vi "Build LV Spec.vi"() -> ()   [LabVIEW 2014]
doc: "This VI will execute a LabVIEW build spec.\n\nArguments:\nLabVIEW project file path\nLabVIEW build spec name\nBuild number"
uses:
  <userlib>/_OpenG.lib/file/file.llb/Convert File Extension (Path)__ogtk.vi
  <vilib>/AppBuilder/AB_API_Simple/Get Build Specification Version (path).vi
  <vilib>/AppBuilder/AB_API_Simple/Set Build Specification Version (path).vi
  <vilib>/AppBuilder/AB_API_Simple/Build (path).vi
  <vilib>/Wiresmith Technology/LabVIEW CLI/CLI Class/CLI.lvclass
  <vilib>/AppBuilder/AB_API_Simple/NI_App_Builder_API.lvlib
panel:
  out "error out":errorcluster
  out "Build Output":path[](array[path])
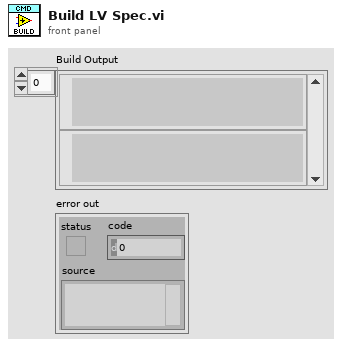
[diagram p1: front panel]
types:
  T1 = typedef "NI_App_Builder_API.lvlib/Build Specification Version.ctl" = cluster{"Major":u16, "Minor":u16, "Fix":u16, "Build":u16}
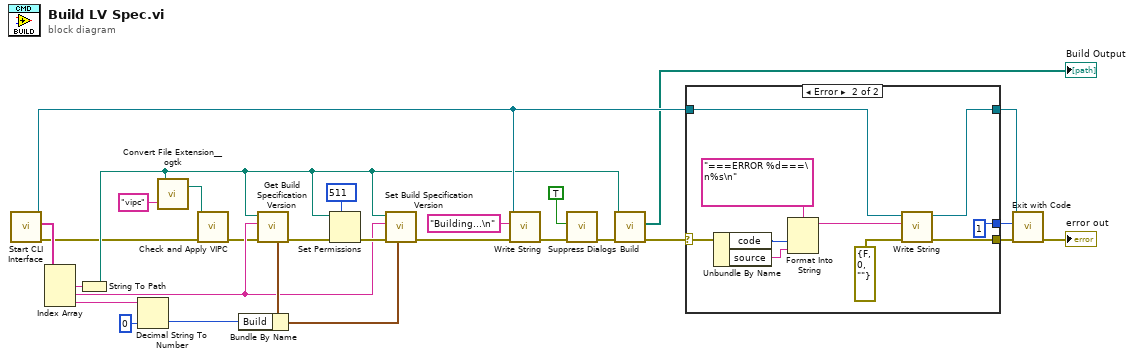
[diagram p0: block diagram]
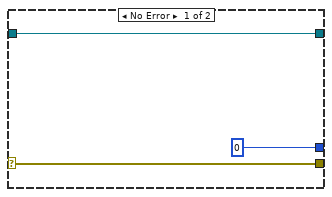
[diagram p2: hidden frame]
diagram:
  n1 = call <vilib>:"Start CLI Interface.vi"() -> ("error out"=w1:errorcluster, "Custom Parameters"=w25:string[], "CLI out"=w22:refnum<class "CLI.lvclass">)  [unwired: 9 in]
  n2 = Index Array(array=w25) -> (element #1=w27:string, element #2=w6:string, element #3=w7:string)  [unwired: 3 in]
  n3 = String To Path(string=w27) -> (path=w2:path)
  n4 = Decimal String To Number(string=w7, default (0L)=u32 0 ("Package Version.build")) -> (number=w26:u32)  [unwired: 1 in, 1 out]
  n5 = call-poly <userlib>:"Convert File Extension__ogtk.vi"("new ending (none)"="vipc", "file name"=w2) -> ("new filename"=w4:path)  [unwired: 1 out]
  n6 = call "Check and Apply VIPC.vi"("error in (no error)"=w1, "VIPC File Path"=w4) -> ("error out"=w3:errorcluster)  [unwired: 9 in]
  n7 = call-poly <vilib>:"Get Build Specification Version.vi"("error in (no error)"=w3, "Name of build specification"=w6, "Path to project"=w2) -> ("error out"=w17:errorcluster, "Build Specification Version"=w9:T1)  [unwired: 7 in]
  n8 = Bundle By Name(cluster=w9, "Build"=w26) -> (w8:T1)
  n9 = Set Permissions(7:i16 511 ("permissions"), 8:w17, 11:w2) -> (0:w16:errorcluster)  [unwired: 2 in, 1 out]
  n10 = call-poly <vilib>:"Set Build Specification Version.vi"("Build Specification Version"=w8, "error in (no error)"=w16, "Name of build specification"=w6, "Path to project"=w2) -> ("error out"=w24:errorcluster)  [unwired: 7 in]
  n11 = call <vilib>:"Write String.vi"("error in (no error)"=w24, "Text to Write"="Building...\n", "CLI in"=w22) -> ("error out"=w14:errorcluster)  [unwired: 7 in, 1 out]
  n12 = call "Suppress Dialogs.vi"("error in (no error)"=w14, "Suppress Dialogs? (F)"=TRUE) -> ("error out"=w13:errorcluster)  [unwired: 9 in]
  n13 = call-poly <vilib>:"Build.vi"("error in (no error)"=w13, "Path to project"=w2) -> ("error out"=w10:errorcluster, "Generated files"=→"Build Output":path[])  [unwired: 8 in]
  n14 = case shown="Error" w10 {
    selector: w10 -> [w31 w38]
    tunnel: w22 -> [w30 w34]
    tunnel: [w31 w37] -> w21
    tunnel: [w30 w36] -> w19
    tunnel: [0 1] -> w20
    frame No Error {
    }
    frame Error {
      n15 = Unbundle By Name(w38) -> ("code"=w39:i32, "source"=w41:string)
      n16 = Format Into String(format string="===ERROR %d===\n%s\n", w39, w41) -> (resulting string=w32:string)  [unwired: 2 in, 1 out]
      n17 = call <vilib>:"Write String.vi"("error in (no error)"=errorcluster {"status"=FALSE, "code"=0, "source"=""} ("error out"), "Text to Write"=w32, "CLI in"=w34) -> ("error out"=w37:errorcluster, "CLI out"=w36:refnum<class "CLI.lvclass">)  [unwired: 7 in]
    }
  }
  n18 = call <vilib>:"Exit with Code.vi"("error in (no error)"=w21, "Exit Code (0)"=w20, "CLI in"=w19) -> ("error out"=→"error out":errorcluster)  [unwired: 8 in]
